vi "Image Processing with Vision Assistant (FPGA) - withDOG.vi"() -> ()   [LabVIEW 2016]
uses:
  <vilib>/visionFPGA/Controls/IMAQ FPGA Image Size.ctl
  <vilib>/rvi/Emulation/niFpgaSctlEmulationGetInTimedLoop.vi
  <vilib>/rvi/Emulation/niFpgaProcessEmulError.vi
  <vilib>/rvi/Emulation/niFpgaGetClockAttributes.vi
  <vilib>/rvi/Emulation/niFpgaEmulationReportErrorSimple.vi
  <vilib>/visionFPGA/Basics/FIFO to Pixel Bus/IMAQ FPGA FIFO to Pixel Bus RGB32x1.vi
  <vilib>/rvi/DataTransferAndStorage/Container/Common/niFpgaContainerGetUniqueNameForEmu.vi
  <vilib>/rvi/DataTransferAndStorage/Container/Common/niFpgaContainerSetEmuInfo.vi
  <vilib>/rvi/eio/common/nirviEmuReportErrorAndStop.vi
  <vilib>/rvi/interface/RandomDataEmulation/niFpgaRandomDataHandleErrors.vi
  <vilib>/rvi/Emulation/niFpgaCriticalErrorInLSC.vi
  <vilib>/rvi/LocalResourceManager/LocalResourceManager.xnode
  <vilib>/rvi/DataTransferAndStorage/Container/XNode/niFpgaContainer.xnode
  <vilib>/rvi/interface/RandomDataEmulation/nirviRandomDataFpgaReadWriteTemplate.vi
  <vilib>/visionFPGA/NI_VDM_FPGA_Basics.lvlib
panel:
  out "Output Valid":bool
  out "Ready For Output":bool=TRUE
  out "StartOfImage":bool=TRUE
  in  "Image Size":T1={"Width"=640, "Height"=480}
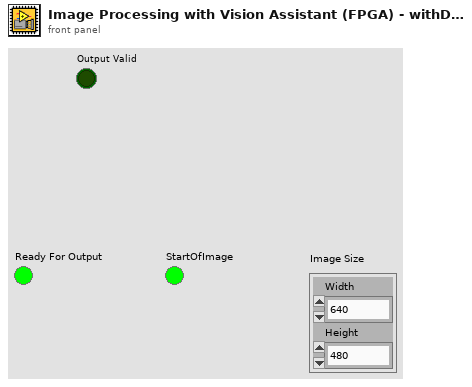
[diagram p1: front panel]
types:
  T1 = typedef "IMAQ FPGA Image Size.ctl" = cluster{"Width":u32, "Height":u32}
  T2 = typedef "IMAQ FPGA Pixel Bus RGB32x1.ctl" = cluster{"Pixel Data":cluster{"A":u8, "R/H":u8, "G/S":u8, "B/L":u8}, "DV":bool, "EOL":bool, "EOI":bool, "Data Type":enum16{"RGB32 x 1"}}
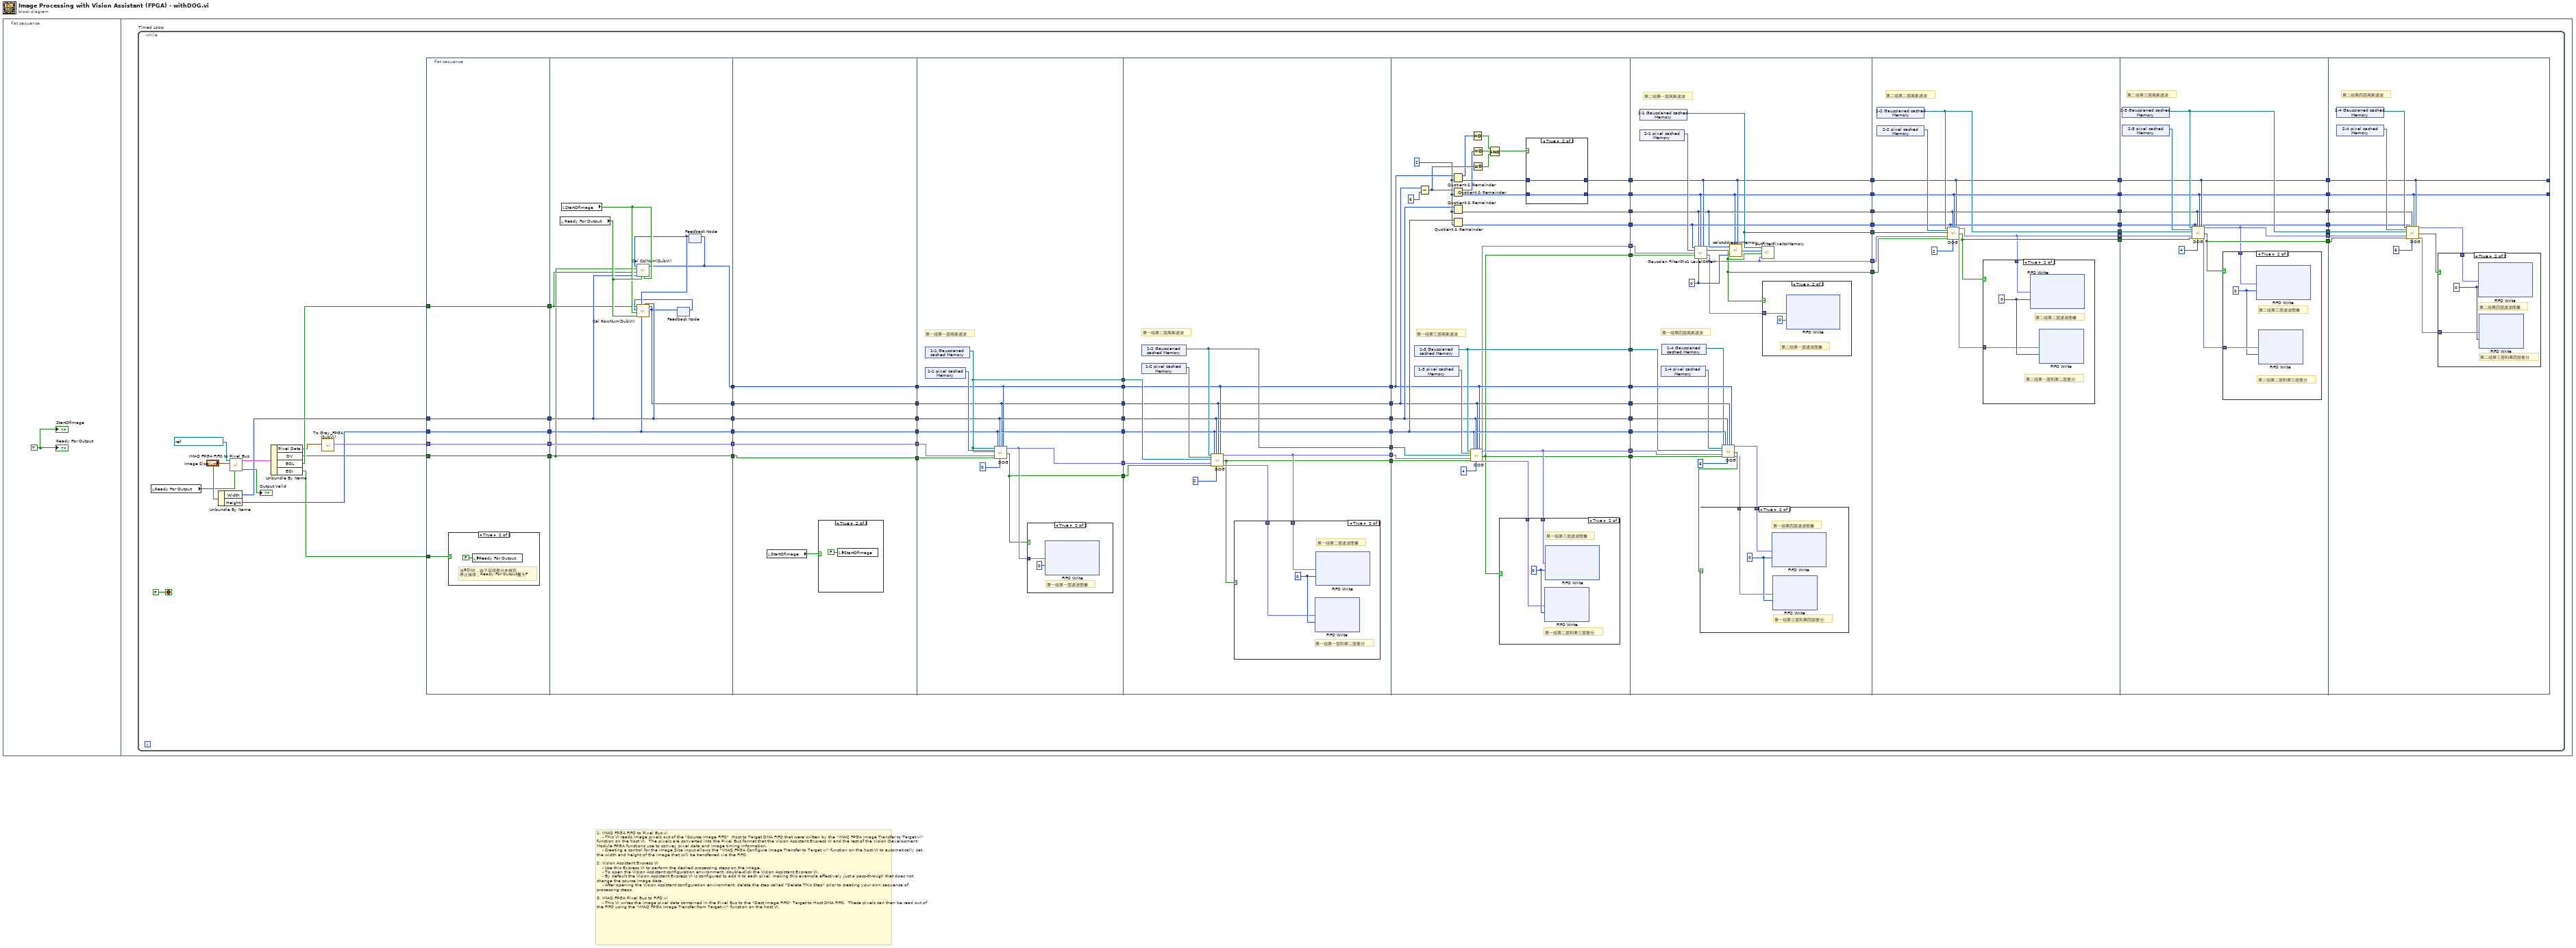
[diagram p0: block diagram]
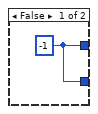
[diagram p6: hidden frame]
diagram:
  # "1. IMAQ FPGA FIFO to Pixel Bus.vi\n    - This VI reads image pixels out of the \"Source Image FIFO\"  Host to Target DMA FIFO that were written by the \"IMAQ FPGA Image Transfer to Target.vi\" function on the host VI.  The pixels are converted into the Pixel Bus format that the Vision Assistant Express VI and the rest of the Vision Development Module FPGA functions use to convey pixel data and image timing information.\n    - Creating a control for the Image Size input allows the \"IMAQ FPGA Configure Image Transfer to Target.vi\" function on the host VI to automatically set the width and height of the image that will be transferred via the FIFO.\n\n2. Vision Assistant Express VI\n    - Use this Express VI to perform the desired processing steps on the image.\n    - To open the Vision Assistant configuration environment, double-click the Vision Assistant Express VI.\n    - By default the Vision Assistant Express VI is configured to add 0 to each pixel, making this example effectively just a pass-through that does not change the source image data.\n    - After opening the Vision Assistant configuration environment, delete the step called \"Delete This Step\" prior to creating your own sequence of processing steps.\n\n3. IMAQ FPGA Pixel Bus to FIFO.vi\n    - This VI writes the image pixel data contained in the Pixel Bus to the \"Dest Image FIFO\" Target to Host DMA FIFO.  These pixels can then be read out of the FIFO using the \"IMAQ FPGA Image Transfer from Target.vi\" function on the host VI."
  n1 = flat-sequence {
    frame #0 {
      w1 = TRUE ("Ready For Output")
      "StartOfImage" <- w1
      "Ready For Output" <- w1
    }
    frame #1 {
      n2 = while "Timed Loop" {
        stop <- FALSE stop-if-true
        n3 = local read "Ready For Output"() -> (w12:bool)
        n4 = Unbundle By Name("Image Size") -> ("Width"=w68:u32, "Height"=w76:u32)
        n5 = call-poly <vilib>:"IMAQ FPGA FIFO to Pixel Bus.vi"("Ready For Output"=w12, "Image Size"="Image Size", "Source Image FIFO"=refnum<k21> "32it Source FIFO") -> ("Output Valid"=→"Output Valid":bool, "Pixel Bus Out"=w78:T2)  [unwired: 6 in, 1 out]
        n6 = Unbundle By Name(w78) -> ("Pixel Data"=w3:cluster{"A":u8, "R/H":u8, "G/S":u8, "B/L":u8}, "DV"=w2:bool, "EOL"=w13:bool, "EOI"=w75:bool)
        n7 = call "To Gray_FPGA (SubVI).vi"("Pixel Data"=w3) -> ("Data Out"=w4:fxp<+,8,8>)  [unwired: 10 in]
        n8 = flat-sequence {
          tunnel: w13 -> [w81]
          tunnel: w75 -> [w80]
          tunnel: w2 -> [w82]
          tunnel: w76 -> [w83]
          tunnel: w68 -> [w84]
          tunnel: w4 -> [w85]
          tunnel: [w85] -> w11
          tunnel: [w84] -> w10
          tunnel: [w83] -> w9
          tunnel: [w82] -> w8
          tunnel: [w81] -> w7
          tunnel: [w89] -> w19
          tunnel: [w87] -> w18
          tunnel: [w97] -> w17
          tunnel: [w94] -> w16
          tunnel: [w91] -> w15
          tunnel: [w92] -> w14
          tunnel: w11 -> [w97]
          tunnel: w10 -> [w94]
          tunnel: w9 -> [w91]
          tunnel: w8 -> [w92]
          tunnel: w7 -> [w93]
          tunnel: [w98] -> w74
          tunnel: [w104] -> w73
          tunnel: [w102] -> w72
          tunnel: [w103] -> w71
          tunnel: [w100] -> w70
          tunnel: [w99] -> w69
          tunnel: w19 -> [w99]
          tunnel: w18 -> [w100]
          tunnel: w17 -> [w104]
          tunnel: w16 -> [w103]
          tunnel: w15 -> [w102]
          tunnel: w14 -> [w98]
          tunnel: w74 -> [w115]
          tunnel: w73 -> [w116]
          tunnel: w72 -> [w111]
          tunnel: w71 -> [w112]
          tunnel: w70 -> [w107]
          tunnel: w69 -> [w106]
          tunnel: [w107] -> w67
          tunnel: [w106] -> w66
          tunnel: [w112] -> w65
          tunnel: [w111] -> w64
          tunnel: [w114] -> w63
          tunnel: [w108] -> w62
          tunnel: [w109] -> w59
          tunnel: w67 -> [w123]
          tunnel: w66 -> [w122]
          tunnel: w65 -> [w126]
          tunnel: w64 -> [w125]
          tunnel: w63 -> [w128]
          tunnel: w62 -> [w127]
          tunnel: [w119] -> w61
          tunnel: [w121] -> w60
          tunnel: w59 -> [w129]
          tunnel: [w123] -> w58
          tunnel: [w122] -> w57
          tunnel: [w126] -> w56
          tunnel: [w125] -> w55
          tunnel: [w124] -> w47
          tunnel: w61 -> [w162]
          tunnel: w60 -> [w161]
          tunnel: w58 -> [w150]
          tunnel: w57 -> [w149]
          tunnel: w56 -> [w155]
          tunnel: w55 -> [w153]
          tunnel: [w137] -> w54
          tunnel: [w135] -> w53
          tunnel: [w150] -> w52
          tunnel: [w149] -> w51
          tunnel: [w155] -> w50
          tunnel: [w153] -> w49
          tunnel: [w159] -> w48
          tunnel: w47 -> [w158]
          tunnel: [w154] -> w46
          tunnel: [w151] -> w45
          tunnel: [w143] -> w44
          tunnel: [w144] -> w43
          tunnel: [w137] -> w42
          tunnel: [w135] -> w41
          tunnel: w54 -> [w193]
          tunnel: w53 -> [w192]
          tunnel: w52 -> [w191]
          tunnel: w51 -> [w190]
          tunnel: w50 -> [w189]
          tunnel: w49 -> [w188]
          tunnel: w48 -> [w185]
          tunnel: w46 -> [w176]
          tunnel: w45 -> [w177]
          tunnel: w44 -> [w175]
          tunnel: w43 -> [w174]
          tunnel: w42 -> [w179]
          tunnel: w41 -> [w180]
          tunnel: [w182] -> w40
          tunnel: [w171] -> w39
          tunnel: [w172] -> w38
          tunnel: [w177] -> w37
          tunnel: [w176] -> w36
          tunnel: [w175] -> w35
          tunnel: [w174] -> w34
          tunnel: w40 -> [w209]
          tunnel: w39 -> [w208]
          tunnel: w38 -> [w207]
          tunnel: w37 -> [w204]
          tunnel: w36 -> [w205]
          tunnel: w35 -> [w203]
          tunnel: w34 -> [w202]
          tunnel: [w206] -> w33
          tunnel: [w202] -> w32
          tunnel: [w203] -> w31
          tunnel: [w205] -> w30
          tunnel: [w204] -> w29
          tunnel: [w199] -> w28
          tunnel: [w201] -> w27
          tunnel: w33 -> [w225]
          tunnel: w32 -> [w221]
          tunnel: w31 -> [w220]
          tunnel: w30 -> [w219]
          tunnel: w29 -> [w218]
          tunnel: w28 -> [w224]
          tunnel: w27 -> [w223]
          tunnel: [w216] -> w26
          tunnel: [w217] -> w25
          tunnel: [w222] -> w24
          tunnel: [w221] -> w23
          tunnel: [w220] -> w22
          tunnel: [w219] -> w21
          tunnel: [w218] -> w20
          tunnel: w26 -> [w240]
          tunnel: w25 -> [w239]
          tunnel: w24 -> [w238]
          tunnel: w23 -> [w235]
          tunnel: w22 -> [w234]
          tunnel: w21 -> [w237]
          tunnel: w20 -> [w236]
          tunnel: [w235] -> _
          tunnel: [w234] -> _
          frame #0 {
            n9 = case shown="True" w80 {
              frame False {
              }
              frame True {
                # "当EOI时，由于后续差分未做完，\n停止接收，Ready For Output置为F"
                n10 = local write "Ready For Output"(FALSE ("Ready For Output")) -> ()
              }
            }
          }
          frame #1 {
            n11 = local read "Ready For Output"() -> (w96:bool)
            n12 = local read "StartOfImage"() -> (w95:bool)
            n13 = feedback #1() -> (w88:u16)  [unwired: 1 in]
            n14 = feedback #2() -> (w90:u16)  [unwired: 1 in]
            n15 = call "Cal ColNum(SubVI).vi"("StartOfImage"=w95, "Ready For Input"=w96, "Width"=w94, "EOL"=w93, "DV"=w92, "curColNum"=w90) -> ("nextColNum"=w87:u16)  [unwired: 5 in]
            n16 = call "Cal RowNum(SubVI).vi"("Width"=w94, "Height"=w91, "curCol"=w90, "Ready For Input"=w96, "startOfImage"=w95, "curRow"=w88, "EOL"=w93) -> ("nextRow"=w89:u16)  [unwired: 4 in]
            n17 = feedback-in #1(w89) -> ()
            n18 = feedback-in #2(w87) -> ()
          }
          frame #2 {
            n19 = local read "StartOfImage"() -> (w101:bool)
            n20 = case shown="True" w101 {
              frame False {
              }
              frame True {
                n21 = local write "StartOfImage"(FALSE ("StartOfImage")) -> ()
              }
            }
          }
          frame #3 {
            # "第一组第一层高斯滤波"
            n22 = xnode "1-1 Gaussianed cached Memory"() -> ("Memory Out"=w109:refnum<k21>)
            n23 = xnode "1-1 pixel cached Memory"() -> ("Memory Out"=w113:refnum<k21>)
            n24 = call "DOG.vi"("Gaussianed cached Memory"=w109, "pixel cached Memory"=w113, "preGaussianed cached Memory"=w109, "Data in"=w116, "DV in"=w115, "Height"=w111, "Width"=w112, "DelayRowCount"=i16 0, "Rows"=w106, "Cols"=w107) -> ("GaussianFilterData out"=w114:fxp<+,12,12>, "DV out"=w108:bool)  [unwired: 7 in, 1 out]
            n25 = case shown="True" w108 {
              tunnel: w114 -> [_ w117]
              frame False {
              }
              frame True {
                # "第一组第一层滤波图像"
                n26 = xnode ("FIFO Write")("Element"=w117, "Timeout"=0) -> ()  [unwired: 1 in, 2 out]
              }
            }
          }
          frame #4 {
            # "第一组第二层高斯滤波"
            n27 = xnode "1-2 Gaussianed cached Memory"() -> ("Memory Out"=w124:refnum<k21>)
            n28 = xnode "1-2 pixel cached Memory"() -> ("Memory Out"=w130:refnum<k21>)
            n29 = call "DOG.vi"("Gaussianed cached Memory"=w124, "pixel cached Memory"=w130, "preGaussianed cached Memory"=w129, "Data in"=w128, "DV in"=w127, "Height"=w125, "Width"=w126, "DelayRowCount"=i16 2, "Rows"=w122, "Cols"=w123) -> ("GaussianFilterData out"=w121:fxp<+,12,12>, "DV out"=w119:bool, "DOG Out"=w120:fxp<+/-,13,13>)  [unwired: 7 in]
            n30 = case shown="True" w119 {
              tunnel: w121 -> [_ w133]
              tunnel: w120 -> [_ w132]
              frame False {
              }
              frame True {
                w134 = 0 ("Timeout")
                # "第一组第一层和第二层差分"
                # "第一组第二层滤波图像"
                n31 = xnode ("FIFO Write")("Element"=w132, "Timeout"=w134) -> ()  [unwired: 1 in, 2 out]
                n32 = xnode ("FIFO Write")("Element"=w133, "Timeout"=w134) -> ()  [unwired: 1 in, 2 out]
              }
            }
          }
          frame #5 {
            w152 = u32 2 ("y")
            # "第一组第三层高斯滤波"
            n33 = xnode "1-3 pixel cached Memory"() -> ("Memory Out"=w160:refnum<k21>)
            n34 = xnode "1-3 Gaussianed cached Memory"() -> ("Memory Out"=w159:refnum<k21>)
            n35 = Subtract(x=w149, y=i16 6) -> (x-y=w140:u16)
            n36 = Quotient & Remainder(x=w150, y=w152) -> (x-y*floor(x/y)=w139:u32, floor(x/y)=w141:u32)
            n37 = Quotient & Remainder(x=w140, y=w152) -> (x-y*floor(x/y)=w138:u32, floor(x/y)=w142:u32)
            n38 = Quotient & Remainder(x=w155, y=w152) -> (floor(x/y)=w154:u32)  [unwired: 1 out]
            n39 = Quotient & Remainder(x=w153, y=w152) -> (floor(x/y)=w151:u32)  [unwired: 1 out]
            n40 = call "DOG.vi"("Gaussianed cached Memory"=w159, "pixel cached Memory"=w160, "preGaussianed cached Memory"=w158, "Data in"=w161, "DV in"=w162, "Height"=w153, "Width"=w155, "DelayRowCount"=i16 4, "Rows"=w149, "Cols"=w150) -> ("GaussianFilterData out"=w137:fxp<+,12,12>, "DV out"=w135:bool, "DOG Out"=w136:fxp<+/-,13,13>)  [unwired: 7 in]
            n41 = Equal To 0?(x=w139) -> (x = 0?=w148:bool)
            n42 = Equal To 0?(x=w138) -> (x = 0?=w147:bool)
            n43 = Greater Or Equal To 0?(x=w140) -> (x >= 0?=w146:bool)
            n44 = Compound Arithmetic op=AND(w148, w147, w146) -> (w145:bool)
            n45 = case shown="True" w135 {
              tunnel: w137 -> [_ w167]
              tunnel: w136 -> [_ w166]
              frame False {
              }
              frame True {
                w168 = 0 ("Timeout")
                # "第一组第二层和第三层差分"
                # "第一组第三层滤波图像"
                n46 = xnode ("FIFO Write")("Element"=w166, "Timeout"=w168) -> ()  [unwired: 1 in, 2 out]
                n47 = xnode ("FIFO Write")("Element"=w167, "Timeout"=w168) -> ()  [unwired: 1 in, 2 out]
              }
            }
            n48 = case shown="True" w145 {
              tunnel: [w163 w165] -> w144
              tunnel: w141 -> [_ w165]
              tunnel: [w163 w164] -> w143
              tunnel: w142 -> [_ w164]
              frame False {
                w163 = i16 -1 ("t")
              }
              frame True {
              }
            }
          }
          frame #6 {
            w173 = i16 0 ("delayRowCount")
            # "第二组第一层高斯滤波"
            # "第一组第四层高斯滤波"
            n49 = xnode "2-1 Gaussianed cached Memory"() -> ("Memory Out"=w182:refnum<k21>)
            n50 = xnode "2-1 pixel cached Memory"() -> ("Memory Out"=w178:refnum<k21>)
            n51 = xnode "1-4 pixel cached Memory"() -> ("Memory Out"=w186:refnum<k21>)
            n52 = xnode "1-4 Gaussianed cached Memory"() -> ("Memory Out"=w187:refnum<k21>)
            n53 = call "Gaussian Filter(Pic1 LevelOther).vi"("Height"=w177, "Width"=w176, "Rows"=w175, "Cols"=w174, "Memory in"=w178, "Data in"=w179, "DV in"=w180, "DelayRowCount"=w173) -> ("DV out"=w172:bool, "Data Out"=w171:fxp<+,8,8>)  [unwired: 6 in]
            n54 = call "DOG.vi"("Gaussianed cached Memory"=w187, "pixel cached Memory"=w186, "preGaussianed cached Memory"=w185, "Data in"=w193, "DV in"=w192, "Height"=w188, "Width"=w189, "DelayRowCount"=i16 6, "Rows"=w190, "Cols"=w191) -> ("GaussianFilterData out"=w181:fxp<+,12,12>, "DV out"=w170:bool, "DOG Out"=w169:fxp<+/-,13,13>)  [unwired: 7 in]
            n55 = case shown="True" w170 {
              tunnel: w181 -> [_ w198]
              tunnel: w169 -> [_ w197]
              frame False {
              }
              frame True {
                w196 = 0 ("Timeout")
                # "第一组第三层和第四层差分"
                # "第一组第四层滤波图像"
                n56 = xnode ("FIFO Write")("Element"=w198, "Timeout"=w196) -> ()  [unwired: 1 in, 2 out]
                n57 = xnode ("FIFO Write")("Element"=w197, "Timeout"=w196) -> ()  [unwired: 1 in, 2 out]
              }
            }
            n58 = call "calcAddressInMemory.vi"("Width"=w176, "Rows"=w175, "delayRowCount"=w173, "Cols"=w174) -> ("addressInMemory"=w183:u16)  [unwired: 5 in]
            n59 = call "putFilterPixeltoMemory.vi"("Data In"=w171, "DV in"=w172, "addressInMemory"=w183, "Memory in"=w182) -> ()
            n60 = case shown="True" w172 {
              tunnel: w171 -> [_ w194]
              frame False {
              }
              frame True {
                # "第二组第一层滤波图像"
                n61 = xnode ("FIFO Write")("Element"=w194, "Timeout"=0) -> ()  [unwired: 1 in, 2 out]
              }
            }
          }
          frame #7 {
            # "第二组第二层高斯滤波"
            n62 = xnode "2-2 Gaussianed cached Memory"() -> ("Memory Out"=w206:refnum<k21>)
            n63 = xnode "2-2 pixel cached Memory"() -> ("Memory Out"=w210:refnum<k21>)
            n64 = call "DOG.vi"("Gaussianed cached Memory"=w206, "pixel cached Memory"=w210, "preGaussianed cached Memory"=w209, "Data in"=w208, "DV in"=w207, "Height"=w204, "Width"=w205, "DelayRowCount"=i16 2, "Rows"=w203, "Cols"=w202) -> ("GaussianFilterData out"=w199:fxp<+,12,12>, "DV out"=w201:bool, "DOG Out"=w200:fxp<+/-,13,13>)  [unwired: 7 in]
            n65 = case shown="True" w201 {
              tunnel: w200 -> [_ w213]
              tunnel: w199 -> [_ w212]
              frame False {
              }
              frame True {
                w214 = 0 ("Timeout")
                # "第二组第一层和第二层差分"
                # "第二组第二层滤波图像"
                n66 = xnode ("FIFO Write")("Element"=w212, "Timeout"=w214) -> ()  [unwired: 1 in, 2 out]
                n67 = xnode ("FIFO Write")("Element"=w213, "Timeout"=w214) -> ()  [unwired: 1 in, 2 out]
              }
            }
          }
          frame #8 {
            # "第二组第三层高斯滤波"
            n68 = xnode "2-3 Gaussianed cached Memory"() -> ("Memory Out"=w222:refnum<k21>)
            n69 = xnode "2-3 pixel cached Memory"() -> ("Memory Out"=w226:refnum<k21>)
            n70 = call "DOG.vi"("Gaussianed cached Memory"=w222, "pixel cached Memory"=w226, "preGaussianed cached Memory"=w225, "Data in"=w224, "DV in"=w223, "Height"=w218, "Width"=w219, "DelayRowCount"=i16 4, "Rows"=w220, "Cols"=w221) -> ("GaussianFilterData out"=w216:fxp<+,12,12>, "DV out"=w217:bool, "DOG Out"=w215:fxp<+/-,13,13>)  [unwired: 7 in]
            n71 = case shown="True" w217 {
              tunnel: w216 -> [_ w230]
              tunnel: w215 -> [_ w229]
              frame False {
              }
              frame True {
                w228 = 0 ("Timeout")
                # "第二组第二层和第三层差分"
                # "第二组第三层滤波图像"
                n72 = xnode ("FIFO Write")("Element"=w230, "Timeout"=w228) -> ()  [unwired: 1 in, 2 out]
                n73 = xnode ("FIFO Write")("Element"=w229, "Timeout"=w228) -> ()  [unwired: 1 in, 2 out]
              }
            }
          }
          frame #9 {
            # "第二组第四层高斯滤波"
            n74 = xnode "2-4 Gaussianed cached Memory"() -> ("Memory Out"=w241:refnum<k21>)
            n75 = xnode "2-4 pixel cached Memory"() -> ("Memory Out"=w242:refnum<k21>)
            n76 = call "DOG.vi"("Gaussianed cached Memory"=w241, "pixel cached Memory"=w242, "preGaussianed cached Memory"=w238, "Data in"=w240, "DV in"=w239, "Height"=w236, "Width"=w237, "DelayRowCount"=i16 6, "Rows"=w234, "Cols"=w235) -> ("GaussianFilterData out"=w232:fxp<+,12,12>, "DV out"=w233:bool, "DOG Out"=w231:fxp<+/-,13,13>)  [unwired: 7 in]
            n77 = case shown="True" w233 {
              tunnel: w232 -> [_ w246]
              tunnel: w231 -> [_ w245]
              frame False {
              }
              frame True {
                w244 = 0 ("Timeout")
                # "第二组第三层和第四层差分"
                # "第二组第四层滤波图像"
                n78 = xnode ("FIFO Write")("Element"=w246, "Timeout"=w244) -> ()  [unwired: 1 in, 2 out]
                n79 = xnode ("FIFO Write")("Element"=w245, "Timeout"=w244) -> ()  [unwired: 1 in, 2 out]
              }
            }
          }
        }
      }
    }
  }
